vi "EditorThumbnail mouseMove.vi"(7 "coordsHorizontal":i32, 8 "error in (no error)":errorcluster, 11 "EditorThumbnail in":refnum<class "EditorThumbnail.lvclass">=refnum) -> (0 "error out":errorcluster, 2 "Timing":bool, 3 "EditorThumbnail out":refnum<class "EditorThumbnail.lvclass">)   [LabVIEW 2018, in "EditorThumbnail.lvclass"]
uses:
  EditorThumbnail.lvclass
  EditorThumbnail.lvclass/EditorThumbnail.ctl
  <vilib>/Utility/miscctls.llb/LVPositionTypeDef.ctl
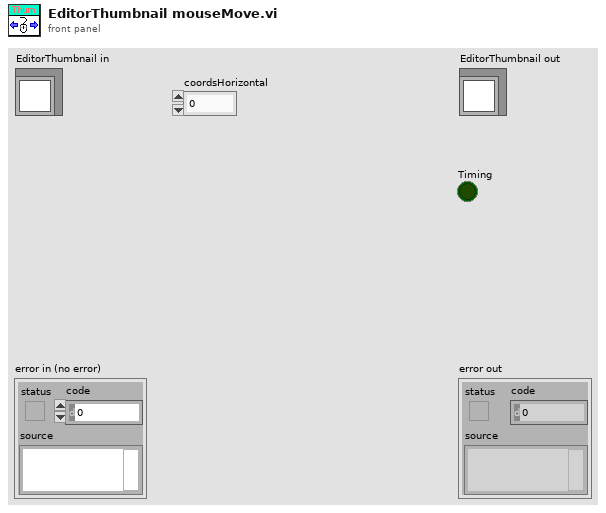
[diagram p1: front panel]
types:
  T1 = typedef "LVPositionTypeDef.ctl" = cluster{"Left":i32, "Top":i32}
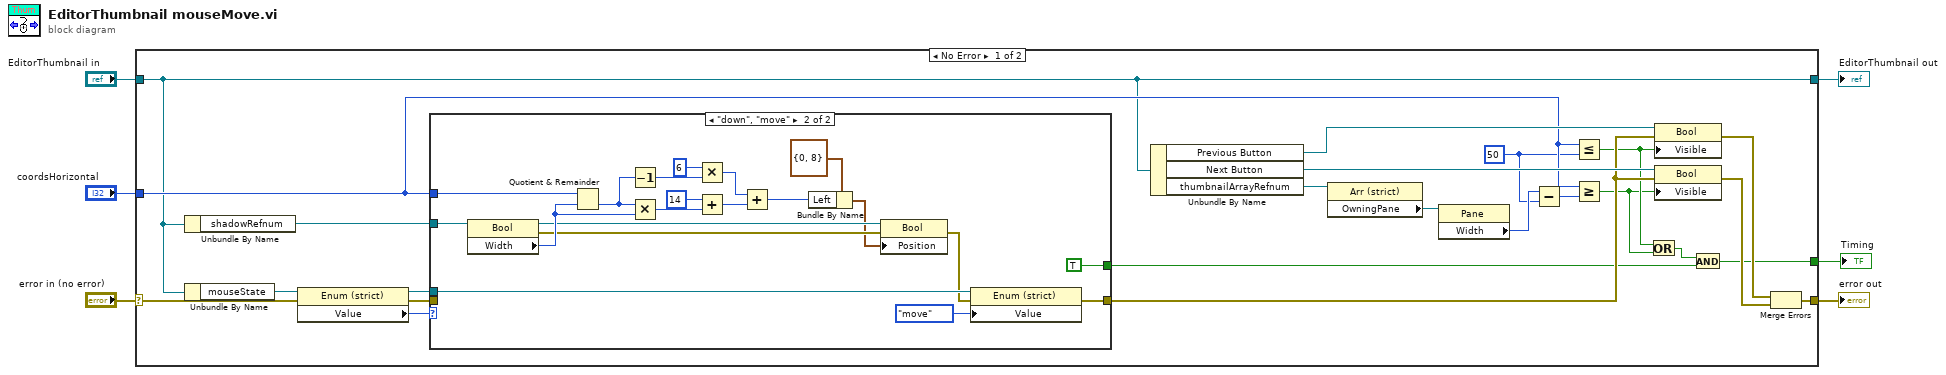
[diagram p0: block diagram]
diagram:
  n1 = case shown="No Error" "error in (no error)" {
    selector: "error in (no error)" -> [w27 w53]
    tunnel: [w13 w53] -> w3
    tunnel: [w10 w52] -> w2
    tunnel: "EditorThumbnail in" -> [w10 w52]
    tunnel: "coordsHorizontal" -> [w20 _]
    tunnel: [w7 _] -> w1
    frame No Error {
      w17 = u32 50 ("Bounds:Area Width")
      n2 = Unbundle By Name(w10) -> ("shadowRefnum"=w25:refnum<vi>)
      n3 = Unbundle By Name(w10) -> ("mouseState"=w30:refnum<vi>)
      n4 = property class="Enum (strict)"(reference=w30, error in=w27) -> (reference out=w28:refnum<vi>, error out=w26:errorcluster, "Value"=w29:enum16{"idle", "down", "move", "up"})
      n5 = case shown="\"down\", \"move\"" w29 {
        tunnel: w28 -> [_ w51]
        tunnel: w26 -> [w31 _]
        tunnel: [w31 w49] -> w16
        tunnel: w25 -> [_ w33]
        tunnel: w20 -> [_ w40]
        tunnel: [_ TRUE] -> w8
        frame Default {
        }
        frame "down", "move" {
          n6 = property class="Bool"(reference=w33) -> (reference out=w39:refnum<vi>, error out=w38:errorcluster, "Width"=w41:u32)  [unwired: 1 in]
          n7 = Quotient & Remainder(x=w40, y=w41) -> (floor(x/y)=w48:u32)  [unwired: 1 out]
          n8 = Decrement(x=w48) -> (x-1=w43:u32)
          n9 = Multiply(x=w48, y=w41) -> (x*y=w47:u32)
          n10 = Multiply(x=u32 6 ("y"), y=w43) -> (x*y=w42:u32)
          n11 = Add(x=u32 14, y=w47) -> (x+y=w45:u32)
          n12 = Add(x=w42, y=w45) -> (x+y=w36:u32)
          n13 = Bundle By Name(cluster=T1 {"Left"=0, "Top"=8} ("Position"), "Left"=w36) -> (w35:T1)
          n14 = property class="Bool"(reference=w39, error in=w38, "Position"=w35) -> (error out=w34:errorcluster)  [unwired: 1 out]
          n15 = property class="Enum (strict)"(reference=w51, error in=w34, "Value"=enum16{"idle", "down", "move", "up"}."move") -> (error out=w49:errorcluster)  [unwired: 1 out]
        }
      }
      n16 = Unbundle By Name(w10) -> ("Previous Button"=w22:refnum<vi>, "Next Button"=w21:refnum<vi>, "thumbnailArrayRefnum"=w24:refnum<vi>)
      n17 = property class="Arr (strict)"(reference=w24) -> ("OwningPane"=w23:refnum<vi>)  [unwired: 1 in, 2 out]
      n18 = property class="Pane"(reference=w23) -> ("Width"=w18:u32)  [unwired: 1 in, 2 out]
      n19 = Subtract(x=w18, y=w17) -> (x-y=w19:u32)
      n20 = Less Or Equal?(x=w20, y=w17) -> (x <= y?=w12:bool)
      n21 = Greater Or Equal?(x=w20, y=w19) -> (x >= y?=w11:bool)
      n22 = Or(x=w12, y=w11) -> (x .or. y?=w9:bool)
      n23 = property class="Bool"(reference=w22, error in=w16, "Visible"=w12) -> (error out=w15:errorcluster)  [unwired: 1 out]
      n24 = property class="Bool"(reference=w21, error in=w16, "Visible"=w11) -> (error out=w14:errorcluster)  [unwired: 1 out]
      n25 = And(x=w9, y=w8) -> (x .and. y?=w7:bool)
      n26 = Merge Errors(w15, w14) -> (w13:errorcluster)
    }
    frame Error {
    }
  }
  "error out" <- w3
  "EditorThumbnail out" <- w2
  "Timing" <- w1
